vi "_Enqueue JKISMQ.vi"(8 "Error in":errorcluster caption="Error in (no error)", 10 "Data":T1, 11 "JKISMQ":T2) -> (0 "Error out":errorcluster, 1 "Target Buzy Error":bool, 3 "JKISMQ":T2)   [LabVIEW 2014, in "JKI-State-Machine-Plus.lvlib"]
uses:
  JKI-State-Machine-Plus.lvlib
  _JKISMQ.ctl
  _Cross JKI StateMachine State Data.ctl
  _Cross JKI StateMachine State Response.ctl
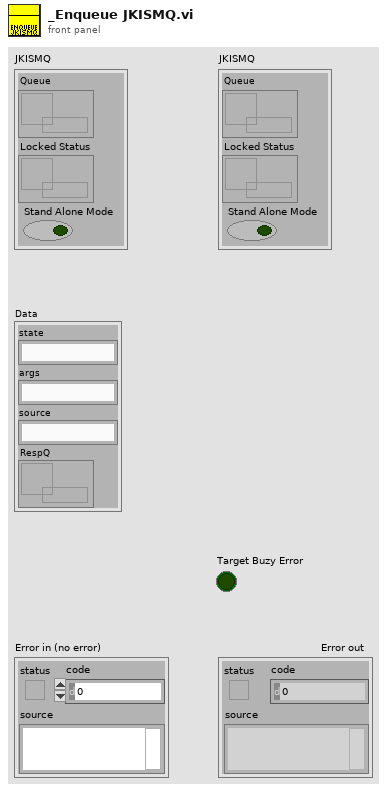
[diagram p1: front panel]
types:
  T1 = typedef "JKI-State-Machine-Plus.lvlib/_Cross JKI StateMachine State Data.ctl" = cluster{"state":string, "args":string, "source":string, "RespQ":refnum<queue>}
  T2 = typedef "JKI-State-Machine-Plus.lvlib/_JKISMQ.ctl" = cluster{"Queue":refnum<queue>, "Locked Status":refnum<data-value>, "Stand Alone Mode":bool}
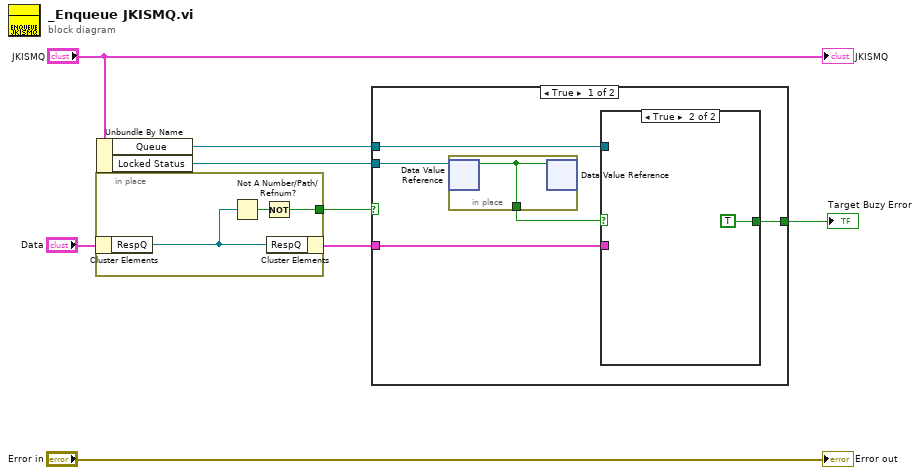
[diagram p0: block diagram]
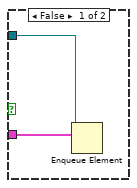
[diagram p2: hidden frame]
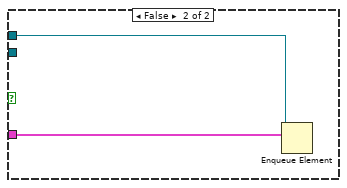
[diagram p3: hidden frame]
diagram:
  n1 = in-place {
    in-place-border: [w9] -> w4
    n2 = in-place-cluster #1("Data") -> ("RespQ"=w11:refnum<queue>)
    n3 = Not A Number/Path/Refnum?(number/path/refnum=w11) -> (NaN/Path/Refnum?=w10:bool)
    n4 = Not(x=w10) -> (.not. x?=w9:bool)
    n5 = in-place-cluster #1("RespQ"=w11) -> (w5:T1)
  }
  n6 = Unbundle By Name("JKISMQ") -> ("Queue"=w6:refnum<queue>, "Locked Status"=w3:refnum<data-value>)
  n7 = case shown="True" w4 {
    tunnel: w6 -> [w16 w22]
    tunnel: w5 -> [w15 w21]
    tunnel: w3 -> [w14 _]
    tunnel: [w12 _] -> w1
    frame True {
      n8 = in-place {
        in-place-border: [w17] -> w13
        n9 = in-place-dvr #2(w14) -> (w17:bool)  [unwired: 1 out]
        n10 = in-place-dvr #2(w17) -> ()  [unwired: 2 out]
      }
      n11 = case shown="True" w13 {
        tunnel: w16 -> [w19 _]
        tunnel: w15 -> [w18 _]
        tunnel: [_ TRUE] -> w12
        frame False {
          n12 = Enqueue Element(queue=w19, element=w18) -> ()  [unwired: 2 in, 3 out]
        }
        frame True {
        }
      }
    }
    frame False {
      n13 = Enqueue Element(queue=w22, element=w21) -> ()  [unwired: 2 in, 3 out]
    }
  }
  "Target Buzy Error" <- w1
  "Error out" <- "Error in"
  "JKISMQ" <- "JKISMQ"
